vi "Untitled 12.vi"() -> ()   [LabVIEW 2012]
uses:
  <vilib>/addons/_office/excel.llb/Excel Get Data (str).vi
  <vilib>/Utility/NIReport.llb/Excel/NI_Excel.lvclass
  <vilib>/Utility/NIReport.llb/NI_report.lvclass
  <vilib>/addons/_office/NI_ReportGenerationToolkit.lvlib
panel:
  out "Numeric 2":i32
  out "Numeric":i32
  in  "start (0, 0)":cluster{"start row":i32, "start column":i32}
  in  "template (empty)":path=path "C:/m100/早車必回-1104.xls"
  out "row":i32
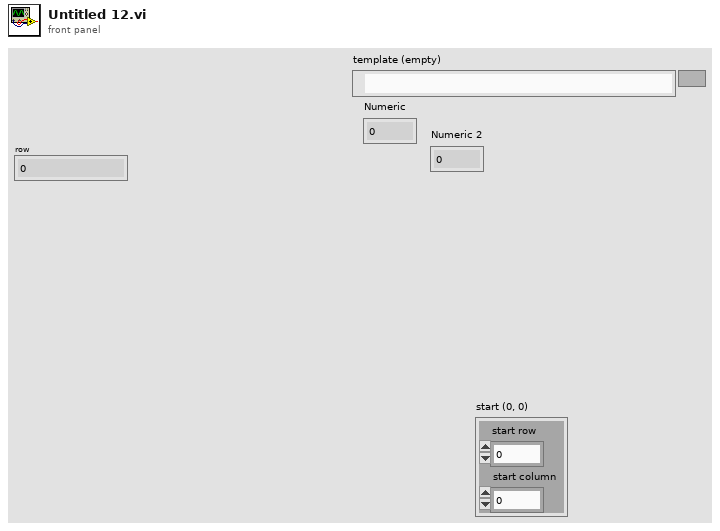
[diagram p1: front panel]
types:
  T1 = enum16{"Standard Report", "HTML", "Word", "Excel"}
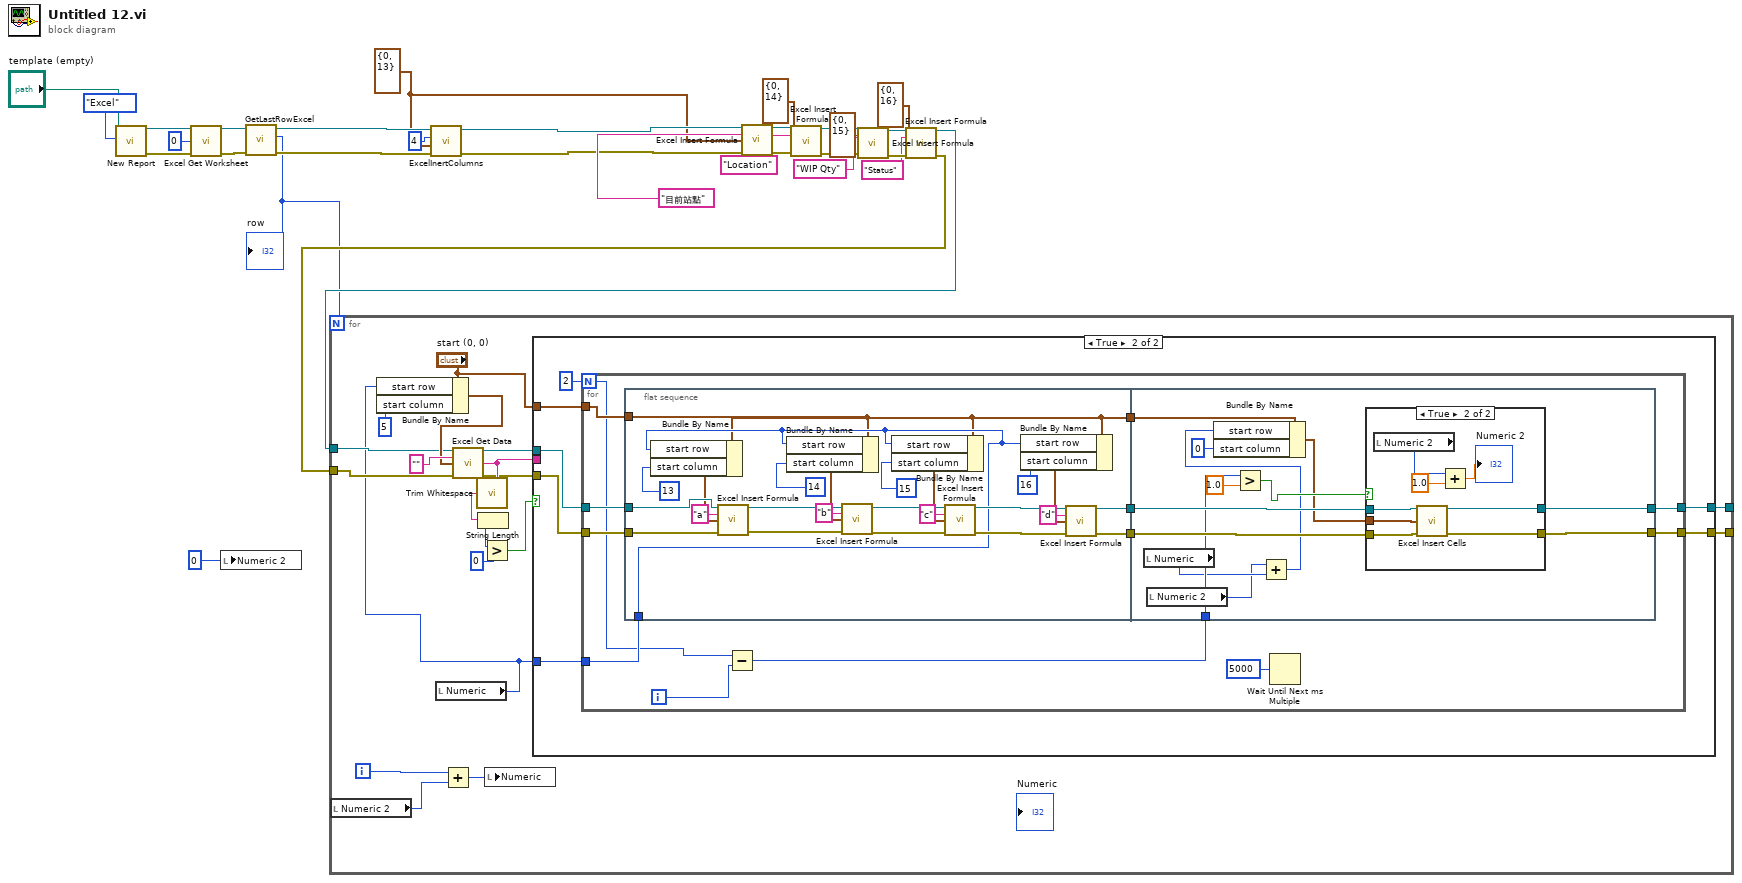
[diagram p0: block diagram]
diagram:
  w7 = cluster{"row":i32, "column":i32} {"row"=0, "column"=13} ("start (0, 0)")
  n1 = call <vilib>:"New Report.vi"("report type"=T1."Excel" ("Report Type"), "template (empty)"="template (empty)") -> ("report out"=w29:refnum<class "NI_report.lvclass">, "error out"=w28:errorcluster)  [unwired: 12 in]
  n2 = call <vilib>:"Excel Get Worksheet.vi"("report in"=w29, "worksheet index (0)"=0, "error in (no error)"=w28) -> ("report out"=w20:refnum<class "NI_report.lvclass">, "error out"=w19:errorcluster)  [unwired: 11 in]
  n3 = local write "Numeric 2"(0) -> ()
  n4 = call "GetLastRowExcel.vi"("error in (no error)"=w19, "report in"=w20) -> ("error out"=w11:errorcluster, "row"=w2:i32, "report out"=w12:refnum<class "NI_report.lvclass">)  [unwired: 7 in]
  "row" <- w2
  n5 = call "ExcelInertColumns.vi"("error in (no error)"=w11, "start (0, 0)"=w7, "Numeric"=4, "report in"=w12) -> ("error out"=w8:errorcluster, "report out"=w9:refnum<class "NI_report.lvclass">)  [unwired: 6 in]
  n6 = call <vilib>:"Excel Insert Formula.vi"("report in"=w9, "formula"="目前站點", "start (0, 0)"=w7, "error in (no error)"=w8) -> ("report out"=w27:refnum<class "NI_report.lvclass">, "error out"=w25:errorcluster)  [unwired: 10 in]
  n7 = call <vilib>:"Excel Insert Formula.vi"("report in"=w27, "formula"="Location", "start (0, 0)"=cluster{"row":i32, "column":i32} {"row"=0, "column"=14}, "error in (no error)"=w25) -> ("report out"=w26:refnum<class "NI_report.lvclass">, "error out"=w24:errorcluster)  [unwired: 10 in]
  n8 = call <vilib>:"Excel Insert Formula.vi"("report in"=w26, "formula"="WIP Qty", "start (0, 0)"=cluster{"row":i32, "column":i32} {"row"=0, "column"=15}, "error in (no error)"=w24) -> ("report out"=w18:refnum<class "NI_report.lvclass">, "error out"=w17:errorcluster)  [unwired: 10 in]
  n9 = call <vilib>:"Excel Insert Formula.vi"("report in"=w18, "formula"="Status", "start (0, 0)"=cluster{"row":i32, "column":i32} {"row"=0, "column"=16}, "error in (no error)"=w17) -> ("report out"=w4:refnum<class "NI_report.lvclass">, "error out"=w3:errorcluster)  [unwired: 10 in]
  n10 = for {
    N: w2 -> [_]
    tunnel: w4 -> [w46]
    tunnel: w3 -> [w45]
    tunnel: [w36] -> _
    tunnel: [w35] -> _
    i -> [w34]
    n11 = local read "Numeric 2"() -> (w33:i32)
    n12 = local read "Numeric"() -> (w31:i32)
    n13 = Bundle By Name(cluster="start (0, 0)", "start row"=w31, "start column"=5) -> (w48:cluster{"start row":i32, "start column":i32})
    n14 = Add(x=w34, y=w33) -> (x+y=w32:i32)
    n15 = call-poly <vilib>:"Excel Get Data.vi"("report in"=w46, "data type"="", "start (0, 0)"=w48, "error in (no error)"=w45) -> ("report out"=w38:refnum<class "NI_report.lvclass">, "data"=w40:string, "error out"=w37:errorcluster)  [unwired: 9 in]
    n16 = call <vilib>:"Trim Whitespace.vi"("string"=w40) -> ("trimmed string"=w43:string)  [unwired: 1 in]
    n17 = String Length(string=w43) -> (length=w42:i32)
    n18 = Greater?(x=w42, y=0) -> (0:w41:bool)
    n19 = local write "Numeric"(w32) -> ()
    n20 = case shown="True" w41 {
      tunnel: w40 -> [_ _]
      tunnel: "start (0, 0)" -> [_ w58]
      tunnel: w38 -> [w51 w57]
      tunnel: w37 -> [w50 w56]
      tunnel: w31 -> [_ w55]
      tunnel: [w51 w53] -> w36
      tunnel: [w50 w52] -> w35
      frame False {
      }
      frame True {
        n21 = for {
          N: 2 -> [w61]
          tunnel: w57 -> [w71]
          tunnel: w55 -> [w70]
          tunnel: [w69] -> w53
          tunnel: w58 -> [w68]
          tunnel: w56 -> [w67]
          tunnel: [w64] -> w52
          i -> [w63]
          n22 = flat-sequence {
            tunnel: w71 -> [w95]
            tunnel: w70 -> [w82]
            tunnel: [w81] -> w66
            tunnel: [w80] -> w65
            tunnel: w68 -> [w72]
            tunnel: w67 -> [w77]
            tunnel: [w72] -> w60
            tunnel: [w105] -> w69
            tunnel: w66 -> [w106]
            tunnel: w65 -> [w104]
            tunnel: [w103] -> w64
            tunnel: w62 -> [w102]
            tunnel: w60 -> [w99]
            frame #0 {
              n23 = Bundle By Name(cluster=w72, "start row"=w82, "start column"=13) -> (w79:cluster{"start row":i32, "start column":i32})
              n24 = call <vilib>:"Excel Insert Formula.vi"("report in"=w95, "formula"="a", "start (0, 0)"=w79, "error in (no error)"=w77) -> ("report out"=w91:refnum<class "NI_report.lvclass">, "error out"=w88:errorcluster)  [unwired: 10 in]
              n25 = Bundle By Name(cluster=w72, "start row"=w82, "start column"=14) -> (w86:cluster{"start row":i32, "start column":i32})
              n26 = call <vilib>:"Excel Insert Formula.vi"("report in"=w91, "formula"="b", "start (0, 0)"=w86, "error in (no error)"=w88) -> ("report out"=w90:refnum<class "NI_report.lvclass">, "error out"=w89:errorcluster)  [unwired: 10 in]
              n27 = Bundle By Name(cluster=w72, "start row"=w82, "start column"=15) -> (w87:cluster{"start row":i32, "start column":i32})
              n28 = call <vilib>:"Excel Insert Formula.vi"("report in"=w90, "formula"="c", "start (0, 0)"=w87, "error in (no error)"=w89) -> ("report out"=w84:refnum<class "NI_report.lvclass">, "error out"=w83:errorcluster)  [unwired: 10 in]
              n29 = Bundle By Name(cluster=w72, "start row"=w82, "start column"=16) -> (w78:cluster{"start row":i32, "start column":i32})
              n30 = call <vilib>:"Excel Insert Formula.vi"("report in"=w84, "formula"="d", "start (0, 0)"=w78, "error in (no error)"=w83) -> ("report out"=w81:refnum<class "NI_report.lvclass">, "error out"=w80:errorcluster)  [unwired: 10 in]
            }
            frame #1 {
              n31 = local read "Numeric"() -> (w101:i32)
              n32 = local read "Numeric 2"() -> (w100:i32)
              n33 = Greater?(x=w102, y=1.0) -> (0:w107:bool)
              n34 = Add(x=w100, y=w101) -> (x+y=w98:i32)
              n35 = Bundle By Name(cluster=w99, "start row"=w98, "start column"=0) -> (w96:cluster{"start row":i32, "start column":i32})
              n36 = case shown="True" w107 {
                tunnel: w106 -> [w110 w118]
                tunnel: [w110 w117] -> w105
                tunnel: w104 -> [w109 w116]
                tunnel: [w109 w115] -> w103
                tunnel: w96 -> [_ w111]
                frame False {
                }
                frame True {
                  n37 = local read "Numeric 2"() -> (w114:i32)
                  n38 = call <vilib>:"Excel Insert Cells.vi"("report in"=w118, "start (0, 0)"=w111, "error in (no error)"=w116) -> ("report out"=w117:refnum<class "NI_report.lvclass">, "error out"=w115:errorcluster)  [unwired: 11 in]
                  n39 = Add(x=w114, y=1.0) -> (x+y=→"Numeric 2":dbl)
                }
              }
            }
          }
          n40 = Subtract(x=w61, y=w63) -> (x-y=w62:i32)
          n41 = Wait Until Next ms Multiple(millisecond multiple=u32 5000) -> ()  [unwired: 1 out]
        }
      }
    }
  }
